vi "SCCSup Dialog - GenMCLB.vi"(4 "online help":T1, 6 "filter parameters":T2, 7 "column header strings":string[](array[string]), 9 "listbox selection mode":i32, 10 "dialog title":string, 11 "complete item names":string[][](array[string])) -> (1 "selection":string[][](array[string]), 3 "cancelled?":bool)   [LabVIEW 2020]
uses:
  <vilib>/SourceControl/support/SCCSup Dialog_GenMCLB_FilterParams.ctl
  <vilib>/SourceControl/support/SCCSup Dialog_GenMCLB_OnlineHelp.ctl
  <vilib>/event_ctls.llb/sizeaction.ctl
  <vilib>/event_ctls.llb/panelstate.ctl
panel:
  out "error out":errorcluster
  in  "error in (no error)":errorcluster
  in  "MC Listbox":i32[](listbox)
  in  "filter":bool=TRUE
  in  "OK":bool
  in  "Cancel":bool
  in  "Help":bool
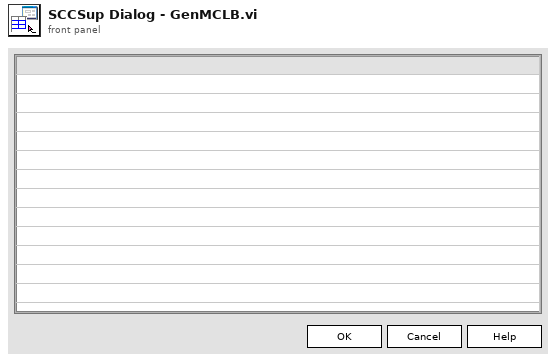
[diagram p1: front panel]
types:
  T1 = typedef "SCCSup Dialog_GenMCLB_OnlineHelp.ctl" = cluster{"Operation":enum16{"Contents", "Key", "Close"}, "String to search for":string, "Path to the help file":path}
  T2 = typedef "SCCSup Dialog_GenMCLB_FilterParams.ctl" = cluster{"checkbox visible?":bool, "boolean text":string, "filter string":string, "filter column":i32}
  T3 = enum32{"invalid OS target", "Mac OS", "Windows 3.1", "Windows 95/NT", "Solaris 1", "Solaris 2", "HP-UX", "PowerMAX", "Linux", "Irix", "Rhapsody", "BeOS", "AIX", "OSF1", "VxWorks", "PharLap", "Carbon", "RTX", "Windows x64", "Linux x64"}
  T4 = typedef "sizeaction.ctl" = enum32{"Minimized", "Maximized", "Resized"}
  T5 = typedef "panelstate.ctl" = enum32{"Standard", "Minimized", "Maximized"}
  T6 = enum32{"Invalid", "Standard", "Closed", "Hidden", "Minimized", "Maximized"}
  T7 = typedef "LVRectTypeDef.ctl" = cluster{"Left":i16, "Top":i16, "Right":i16, "Bottom":i16}
  T8 = enum32{"invalid OS target", "Mac OS", "Windows 3.1", "Windows 95/NT", "Solaris 1", "Solaris 2", "HP-UX", "PowerMAX", "Linux", "Irix", "Rhapsody", "BeOS", "AIX", "OSF1", "VxWorks", "PharLap", "Carbon", "RTX", "Windows x64", "Linux x64", "Mac OS X x64"}
  T9 = typedef "LVPoint32TypeDef.ctl" = cluster{"Horizontal":i32, "Vertical":i32}
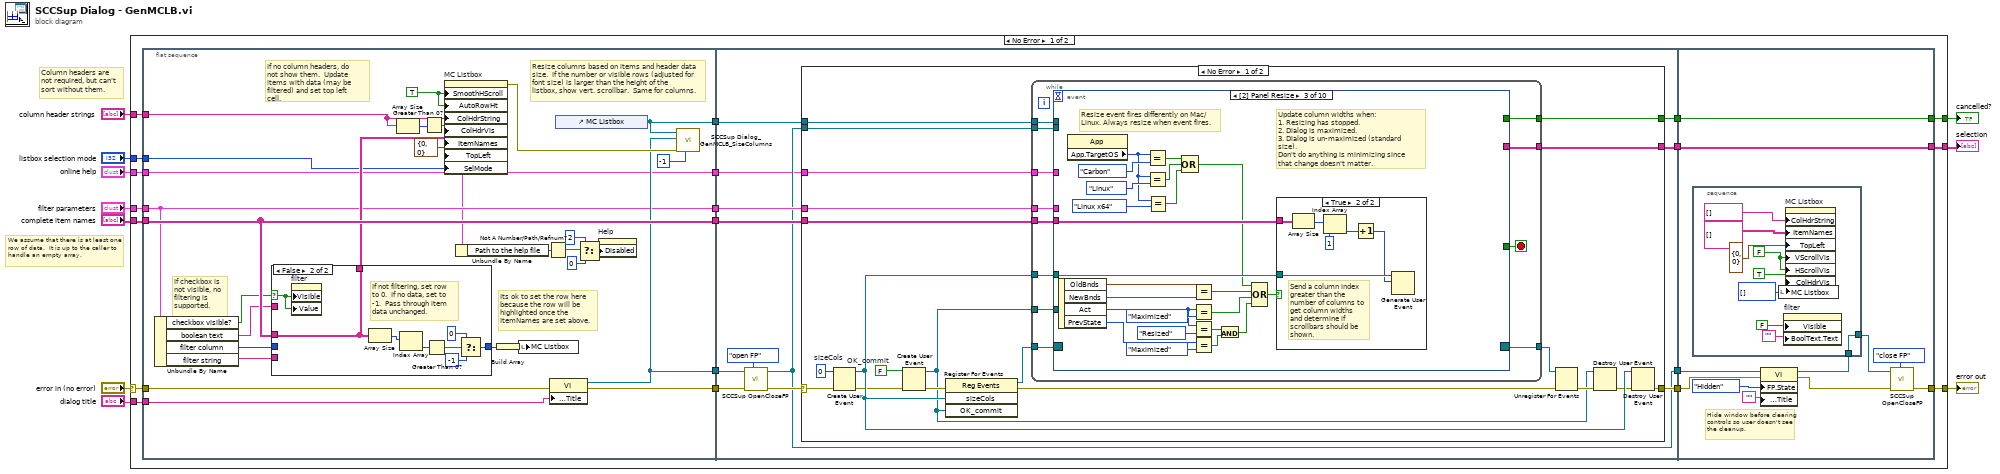
[diagram p0: block diagram]
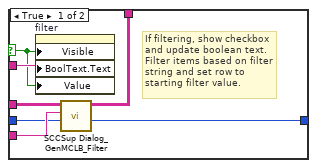
[diagram p2: hidden frame]
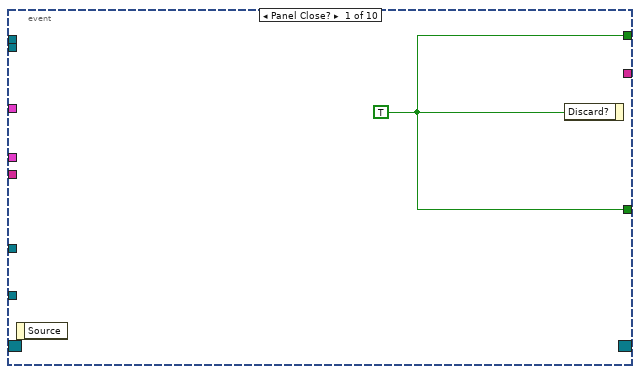
[diagram p3: hidden frame]
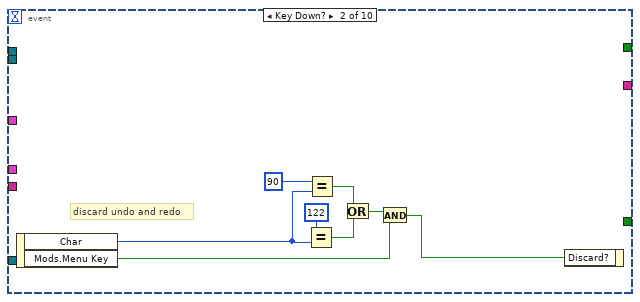
[diagram p4: hidden frame]
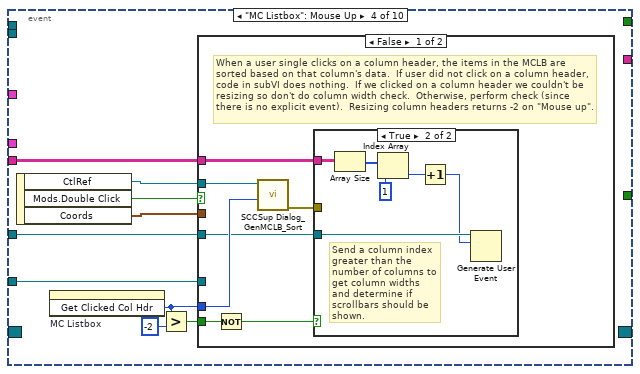
[diagram p6: hidden frame]
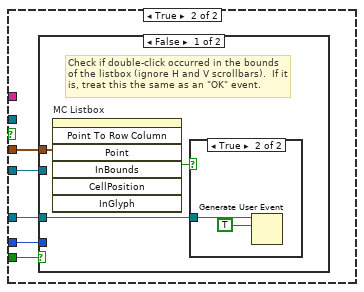
[diagram p8: hidden frame]
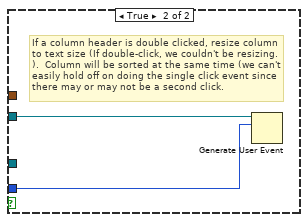
[diagram p10: hidden frame]
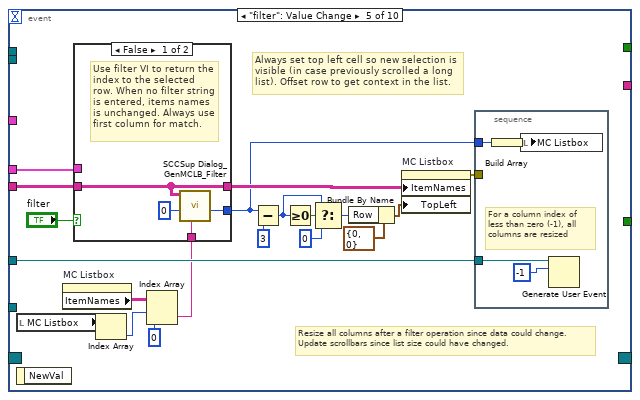
[diagram p11: hidden frame]
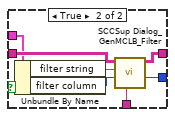
[diagram p12: hidden frame]
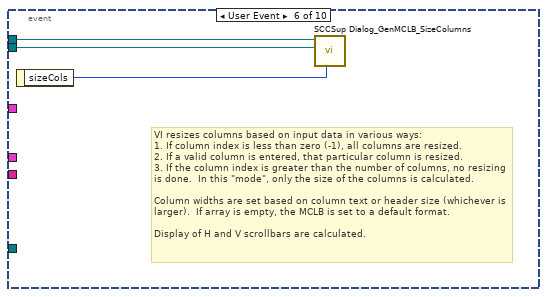
[diagram p13: hidden frame]
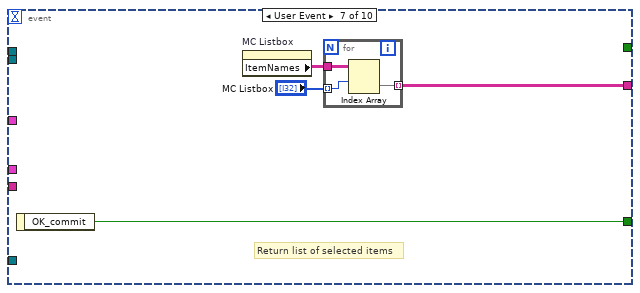
[diagram p14: hidden frame]
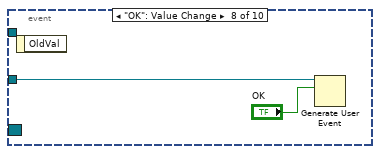
[diagram p15: hidden frame]
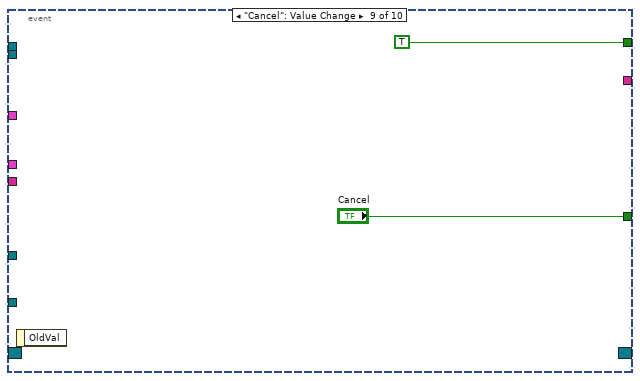
[diagram p16: hidden frame]
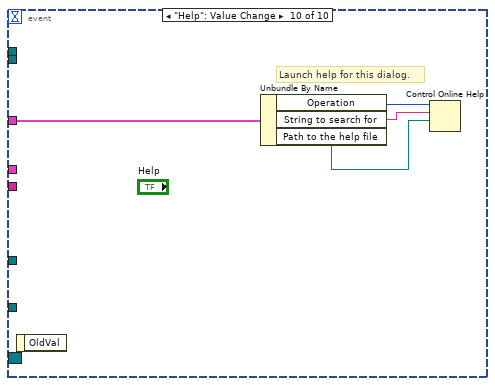
[diagram p17: hidden frame]
diagram:
  # "Column headers are not required, but can't sort without them."
  # "We assume that there is at least one row of data.  It is up to the caller to handle an empty array."
  n1 = case shown="No Error" "error in (no error)" {
    selector: "error in (no error)" -> [w16 w263]
    tunnel: "dialog title" -> [w23 _]
    tunnel: "complete item names" -> [w22 _]
    tunnel: "column header strings" -> [w21 _]
    tunnel: "filter parameters" -> [w20 _]
    tunnel: "listbox selection mode" -> [w19 _]
    tunnel: [w18 _] -> w5
    tunnel: [w17 _] -> w4
    tunnel: [w13 w263] -> w2
    tunnel: "online help" -> [w12 _]
    frame No Error {
      n2 = flat-sequence {
        tunnel: [w45] -> w30
        tunnel: w23 -> [w58]
        tunnel: w22 -> [w53]
        tunnel: w21 -> [w54]
        tunnel: [w53] -> w29
        tunnel: w20 -> [w41]
        tunnel: [w41] -> w28
        tunnel: [w47] -> w27
        tunnel: w19 -> [w46]
        tunnel: w16 -> [w44]
        tunnel: [w43] -> w15
        tunnel: w12 -> [w36]
        tunnel: [w36] -> w11
        tunnel: [w75] -> w26
        tunnel: w30 -> [w84]
        tunnel: w29 -> [w83]
        tunnel: w28 -> [w82]
        tunnel: w27 -> [w81]
        tunnel: [w80] -> w25
        tunnel: [w79] -> w24
        tunnel: w15 -> [w78]
        tunnel: [w76] -> w14
        tunnel: w11 -> [w74]
        tunnel: w26 -> [w253]
        tunnel: [w251] -> w18
        tunnel: w25 -> [w251]
        tunnel: [w250] -> w17
        tunnel: w24 -> [w250]
        tunnel: w14 -> [w249]
        tunnel: [w247] -> w13
        frame #0 {
          w42 = TRUE ("Smooth Horizontal Scrolling")
          # "If checkbox is not visible, no filtering is supported."
          # "Resize columns based on items and header data size.  If the number or visible rows (adjusted for font size) is larger than the height of the listbox, show vert. scrollbar.  Same for columns."
          # "Its ok to set the row here because the row will be highlighted once the ItemNames are set above."
          # "If no column headers, do not show them.  Update items with data (may be filtered) and set top left cell."
          n3 = Unbundle By Name(w41) -> ("checkbox visible?"=w40:bool, "boolean text"=w39:string, "filter column"=w38:i32, "filter string"=w37:string)
          n4 = case shown="False" w40 {
            selector: w40 -> [w59 w66]
            tunnel: w39 -> [w65 _]
            tunnel: w53 -> [w64 w68]
            tunnel: w38 -> [w61 _]
            tunnel: w37 -> [w62 _]
            tunnel: [w60 w69] -> w57
            tunnel: [w63 w68] -> w51
            frame True {
              # "If filtering, show checkbox and update boolean text.  Filter items based on filter string and set row to starting filter value."
              n5 = property on="filter" class="Bool (strict)"("Visible"=w59, "BoolText.Text"=w65, "Value"=w59) -> ()  [unwired: 2 in, 2 out]
              n6 = call <vilib>:"SCCSup Dialog_GenMCLB_Filter.vi"("filter column"=w61, "filter string"=w62, "complete item names"=w64) -> ("filter string row index"=w60:i32, "filtered item names"=w63:string[][])  [unwired: 7 in]
            }
            frame False {
              # "If not filtering, set row to 0.  If no data, set to -1.  Pass through item data unchanged."
              n7 = property on="filter" class="Bool (strict)"("Visible"=w66, "Value"=w66) -> ()  [unwired: 2 in, 2 out]
              n8 = Array Size(array=w68) -> (size(s)=w73:i32[])
              n9 = Index Array(array=w73) -> (element=w71:i32)  [unwired: 1 in]
              n10 = Greater Than 0?(x=w71) -> (x > 0?=w72:bool)
              n11 = Select(t=0, s=w72, f=-1 ("index of element")) -> (s? t:f=w69:i32)
            }
          }
          n12 = Array Size(array=w54) -> (size(s)=w56:i32)
          n13 = Greater Than 0?(x=w56) -> (x > 0?=w55:bool)
          n14 = property on="MC Listbox" class="MCListbox (strict)"("SmoothHScroll"=w42, "AutoRowHt"=w42, "ColHdrString"=w54, "ColHdrVis"=w55, "ItemNames"=w51, "TopLeft"=cluster{"Row":u32, "Column":u32} {"Row"=0, "Column"=0} ("Top Left Visible Cell"), "SelMode"=w46) -> (error out=w49:errorcluster)  [unwired: 2 in, 1 out]
          n15 = Unbundle By Name(w36) -> ("Path to the help file"=w35:path)
          n16 = Build Array(w57) -> (w48:i32[])
          n17 = local write "MC Listbox"(w48) -> ()
          n18 = Not A Number/Path/Refnum?(number/path/refnum=w35) -> (NaN/Path/Refnum?=w34:bool)
          n19 = property class="VI"(error in=w44, "Front Panel.Title"=w58) -> (reference out=w45:refnum<vi>, error out=w43:errorcluster)  [unwired: 1 in]
          n20 = control-ref of="MC Listbox"() -> (w47:refnum<vi>)
          n21 = Select(t=u8 2 ("Disabled"), s=w34, f=u8 0 ("Disabled")) -> (s? t:f=w31:u8)
          n22 = property on="Help" class="Bool"("Disabled"=w31) -> ()  [unwired: 2 in, 2 out]
          n23 = call <vilib>:"SCCSup Dialog_GenMCLB_SizeColumns.vi"("column index"=-1, "error in (no error)"=w49, "VI Refnum"=w45, "Multicolumn Listbox"=w47) -> ()  [unwired: 6 in, 2 out]
        }
        frame #1 {
          n24 = call <vilib>:"SCCSup OpenCloseFP.vi"("function"=enum16{"open FP", "close FP"}."open FP", "error in (no error)"=w78, "VI Refnum in"=w84) -> ("error out"=w77:errorcluster, "VI Refnum out"=w75:refnum<vi>)  [unwired: 7 in]
          n25 = case shown="No Error" w77 {
            selector: w77 -> [w100 w242]
            tunnel: w75 -> [w94 _]
            tunnel: w83 -> [w105 _]
            tunnel: w82 -> [w104 _]
            tunnel: w81 -> [w103 _]
            tunnel: [w102 _] -> w80
            tunnel: [w101 _] -> w79
            tunnel: [w95 w242] -> w76
            tunnel: w74 -> [w86 _]
            frame No Error {
              w90 = FALSE  # OK_commit
              w93 = 0  # sizeCols
              n26 = Create User Event(user event datatype=w93, error in=w100) -> (user event=w96:refnum<user-event>, error out=w91:errorcluster)
              n27 = Create User Event(user event datatype=w90, error in=w91) -> (user event=w87:refnum<user-event>, error out=w92:errorcluster)
              n28 = register-events(error in=w92, w96, w87) -> (reference out=w99:refnum<event-registration>, error out=w98:errorcluster)  [unwired: 1 in]
              n29 = while {
                tunnel: [w116] -> w102
                tunnel: w94 -> [w111]
                tunnel: [w115] -> w101
                tunnel: w105 -> [w114]
                tunnel: w104 -> [w113]
                tunnel: w103 -> [w112]
                tunnel: w96 -> [w108]
                tunnel: w99 -> [w110]
                tunnel: [w109] -> w97
                tunnel: w87 -> [w107]
                tunnel: w86 -> [w106]
                stop <- w117 stop-if-true
                n30 = event shown="[2] Panel Resize" {
                  selector: w110 -> [_ _ _ _ _ _ _ _ _ _]
                  dyn-events: [_ _ _ _ _ _ _ _ _ _] -> w109
                  timeout: _ -> [_ _ _ _ _ _ _ _ _ _]
                  tunnel: [w118 _ _ _ _ _ w227 _ "Cancel" _] -> w117
                  tunnel: [w118 _ _ _ _ _ _ _ TRUE _] -> w116
                  tunnel: [_ _ _ _ _ _ w228 _ _ _] -> w115
                  tunnel: w114 -> [_ _ w136 w159 w208 _ _ _ _ _]
                  tunnel: w113 -> [_ _ _ _ w206 _ _ _ _ _]
                  tunnel: w112 -> [_ _ _ _ _ w226 _ _ _ _]
                  tunnel: w111 -> [_ _ _ _ _ w225 _ _ _ _]
                  tunnel: w108 -> [_ _ w137 w158 w204 _ _ _ _ _]
                  tunnel: w107 -> [_ _ _ w157 _ _ _ w235 _ _]
                  tunnel: w106 -> [_ _ _ _ _ _ _ _ _ w238]
                  event Panel Close? {
                    w118 = TRUE
                    n31 = event-data() -> ()  [unwired: 1 in, 1 out]
                    n32 = event-data("Discard?"=w118) -> ()  [unwired: 1 in, 1 out]
                  }
                  event Key Down? {
                    # "discard undo and redo"
                    n33 = event-data() -> ("Char"=w121:i16, "Mods.Menu Key"=w120:bool)  [unwired: 1 in]
                    n34 = Equal?(x=i16 122, y=w121) -> (x = y?=w124:bool)
                    n35 = Equal?(x=i16 90, y=w121) -> (x = y?=w123:bool)
                    n36 = Or(x=w123, y=w124) -> (x .or. y?=w122:bool)
                    n37 = And(x=w122, y=w120) -> (x .and. y?=w119:bool)
                    n38 = event-data("Discard?"=w119) -> ()  [unwired: 1 in, 1 out]
                  }
                  event Panel Resize {
                    # "Resize event fires differently on Mac/Linux. Always resize when event fires."
                    # "Update column widths when:\n1. Resizing has stopped.\n2. Dialog is maximized.\n3. Dialog is un-maximized (standard size).\nDon't do anything is minimizing since that change doesn't matter."
                    n39 = event-data() -> ("OldBnds"=w149:T7, "NewBnds"=w148:T7, "Act"=w142:T4, "PrevState"=w144:T5)  [unwired: 1 in]
                    n40 = property class="App"() -> ("App.TargetOS"=w129:T8)  [unwired: 2 in, 2 out]
                    n41 = Equal?(x=w129, y=T3."Carbon" ("Application:Target:Operating System")) -> (x = y?=w135:bool)
                    n42 = Equal?(x=w129, y=T3."Linux" ("Application:Target:Operating System")) -> (x = y?=w130:bool)
                    n43 = Equal?(x=w129, y=T3."Linux x64" ("Application:Target:Operating System")) -> (x = y?=w127:bool)
                    n44 = Compound Arithmetic op=OR(w135, w130, w127) -> (w134:bool)
                    n45 = Equal?(x=w149, y=w148) -> (x = y?=w133:bool)
                    n46 = Equal?(x=w142, y=sizeaction."Maximized") -> (x = y?=w145:bool)
                    n47 = Equal?(x=w142, y=sizeaction."Resized") -> (x = y?=w140:bool)
                    n48 = Equal?(x=w144, y=panelstate."Maximized" ("PrevState")) -> (x = y?=w139:bool)
                    n49 = And(x=w140, y=w139) -> (x .and. y?=w138:bool)
                    n50 = Compound Arithmetic op=OR(w134, w133, w145, w138) -> (w146:bool)
                    n51 = case shown="True" w146 {
                      tunnel: w137 -> [_ w155]
                      tunnel: w136 -> [_ w151]
                      frame False {
                      }
                      frame True {
                        # "Send a column index greater than the number of columns to get column widths and determine if scrollbars should be shown."
                        n52 = Array Size(array=w151) -> (size(s)=w153:i32[])
                        n53 = Index Array(array=w153, index=1) -> (element=w154:i32)
                        n54 = Increment(x=w154) -> (x+1=w150:i32)
                        n55 = Generate User Event(user event=w155, event data cluster=w150) -> ()  [unwired: 2 in, 2 out]
                      }
                    }
                  }
                  event "MC Listbox": Mouse Up {
                    n56 = event-data() -> ("CtlRef"=w163:refnum<vi>, "Mods.Double Click"=w164:bool, "Coords"=w156:T9)  [unwired: 1 in]
                    n57 = invoke on="MC Listbox" class="MCListbox (strict)" method="Get Clicked Col Hdr"() -> ("Get Clicked Column Header"=w161:i32)  [unwired: 3 in, 2 out]
                    n58 = Greater?(x=w161, y=-2) -> (0:w160:bool)
                    n59 = case shown="False" w164 {
                      tunnel: w163 -> [w169 _]
                      tunnel: w161 -> [w171 w182]
                      tunnel: w160 -> [w170 w181]
                      tunnel: w159 -> [w168 _]
                      tunnel: w158 -> [w166 w180]
                      tunnel: w157 -> [_ w179]
                      tunnel: w156 -> [_ w178]
                      frame False {
                        # "When a user single clicks on a column header, the items in the MCLB are sorted based on that column's data.  If user did not click on a column header, code in subVI does nothing.  If we clicked on a column header we couldn't be resizing so don't do column width check.  Otherwise, perform check (since there is no explicit event).  Resizing column headers returns -2 on \"Mouse up\"."
                        n60 = Not(x=w170) -> (.not. x?=w167:bool)
                        n61 = call <vilib>:"SCCSup Dialog_GenMCLB_Sort.vi"("Clicked Col Hdr"=w171, "MCListbox Refnum"=w169) -> ("error out"=w165:errorcluster)  [unwired: 9 in]
                        n62 = case shown="True" w167 {
                          tunnel: w168 -> [_ w177]
                          tunnel: w166 -> [_ w173]
                          tunnel: w165 -> [_ _]
                          frame False {
                          }
                          frame True {
                            # "Send a column index greater than the number of columns to get column widths and determine if scrollbars should be shown."
                            n63 = Array Size(array=w177) -> (size(s)=w175:i32[])
                            n64 = Index Array(array=w175, index=1) -> (element=w174:i32)
                            n65 = Increment(x=w174) -> (x+1=w172:i32)
                            n66 = Generate User Event(user event=w173, event data cluster=w172) -> ()  [unwired: 2 in, 2 out]
                          }
                        }
                      }
                      frame True {
                        n67 = case shown="False" w181 {
                          tunnel: w182 -> [_ w188]
                          tunnel: w180 -> [_ w189]
                          tunnel: w179 -> [w183 _]
                          tunnel: w178 -> [w185 _]
                          frame False {
                            # "Check if double-click occurred in the bounds of the listbox (ignore H and V scrollbars).  If it is, treat this the same as an \"OK\" event."
                            n68 = invoke on="MC Listbox" class="MCListbox (strict)" method="Point To Row Column"("Point"=w185) -> ("InBounds"=w184:bool)  [unwired: 6 in, 6 out]
                            n69 = case shown="True" w184 {
                              tunnel: w183 -> [_ w187]
                              frame False {
                              }
                              frame True {
                                n70 = Generate User Event(user event=w187, event data cluster=TRUE ("event data")) -> ()  [unwired: 2 in, 2 out]
                              }
                            }
                          }
                          frame True {
                            # "If a column header is double clicked, resize column to text size (If double-click, we couldn't be resizing.).  Column will be sorted at the same time (we can't easily hold off on doing the single click event since there may or may not be a second click."
                            n71 = Generate User Event(user event=w189, event data cluster=w188) -> ()  [unwired: 2 in, 2 out]
                          }
                        }
                      }
                    }
                  }
                  event "filter": Value Change {
                    # "Always set top left cell so new selection is visible (in case previously scrolled a long list). Offset row to get context in the list."
                    # "Resize all columns after a filter operation since data could change.  Update scrollbars since list size could have changed."
                    n72 = local read "MC Listbox"() -> (w196:i32[])
                    n73 = event-data() -> ()  [unwired: 1 in, 1 out]
                    n74 = property on="MC Listbox" class="MCListbox (strict)"() -> ("ItemNames"=w197:string[][])  [unwired: 2 in, 2 out]
                    n75 = Index Array(array=w196) -> (element=w195:i32)  [unwired: 1 in]
                    n76 = Index Array(array=w197, index (row)=w195, index (col)=0 ("disabled index (col)")) -> (element=w193:string)
                    n77 = case shown="False" "filter" {
                      tunnel: w208 -> [w214 w223]
                      tunnel: [w214 w222] -> w207
                      tunnel: [w215 w221] -> w192
                      tunnel: w206 -> [_ w220]
                      tunnel: w193 -> [w216 w217]
                      frame False {
                        # "Use filter VI to return the index to the selected row. When no filter string is entered, items names is unchanged. Always use first column for match."
                        n78 = call <vilib>:"SCCSup Dialog_GenMCLB_Filter.vi"("current selection"=w216, "filter column"=0, "complete item names"=w214) -> ("filter string row index"=w215:i32)  [unwired: 7 in, 1 out]
                      }
                      frame True {
                        n79 = Unbundle By Name(w220) -> ("filter string"=w219:string, "filter column"=w218:i32)
                        n80 = call <vilib>:"SCCSup Dialog_GenMCLB_Filter.vi"("current selection"=w217, "filter column"=w218, "filter string"=w219, "complete item names"=w223) -> ("filter string row index"=w221:i32, "filtered item names"=w222:string[][])  [unwired: 6 in]
                      }
                    }
                    n81 = Subtract(x=w192, y=3) -> (x-y=w190:i32)
                    n82 = Greater Or Equal To 0?(x=w190) -> (x >= 0?=w203:bool)
                    n83 = Select(t=w190, s=w203, f=0 ("y")) -> (s? t:f=w200:i32)
                    n84 = Bundle By Name(cluster=cluster{"Row":u32, "Column":u32} {"Row"=0, "Column"=0} ("Top Left Visible Cell"), "Row"=w200) -> (w199:cluster{"Row":u32, "Column":u32})
                    n85 = property on="MC Listbox" class="MCListbox (strict)"("ItemNames"=w207, "TopLeft"=w199) -> (error out=w198:errorcluster)  [unwired: 2 in, 1 out]
                    n86 = stacked-sequence {
                      tunnel: w204 -> [w211]
                      tunnel: w198 -> [_]
                      tunnel: w192 -> [w209]
                      frame #0 {
                        # "For a column index of less than zero (-1), all columns are resized"
                        n87 = Build Array(w209) -> (w212:i32[])
                        n88 = local write "MC Listbox"(w212) -> ()
                        n89 = Generate User Event(user event=w211, event data cluster=-1 ("column index")) -> ()  [unwired: 2 in, 2 out]
                      }
                    }
                  }
                  event User Event {
                    # "VI resizes columns based on input data in various ways:\n1. If column index is less than zero (-1), all columns are resized.\n2. If a valid column is entered, that particular column is resized.\n3. If the column index is greater than the number of columns, no resizing is done.  In this \"mode\", only the size of the columns is calculated.\n\nColumn widths are set based on column text or header size (whichever is larger).  If array is empty, the MCLB is set to a default format.\n\nDisplay of H and V scrollbars are calculated."
                    n90 = event-data() -> ("sizeCols"=w224:i32)  [unwired: 1 in]
                    n91 = call <vilib>:"SCCSup Dialog_GenMCLB_SizeColumns.vi"("column index"=w224, "VI Refnum"=w225, "Multicolumn Listbox"=w226) -> ()  [unwired: 7 in, 2 out]
                  }
                  event User Event {
                    # "Return list of selected items"
                    n92 = event-data() -> ("OK_commit"=w227:bool)  [unwired: 1 in]
                    n93 = property on="MC Listbox" class="MCListbox (strict)"() -> ("ItemNames"=w230:string[][])  [unwired: 2 in, 2 out]
                    n94 = for {
                      tunnel: w230 -> [w233]
                      tunnel: [w232] -> w228 mode=indexing
                      tunnel: "MC Listbox" -> [w231] mode=indexing
                      n95 = Index Array(array=w233, index (row)=w231) -> (element=w232:string[])  [unwired: 1 in]
                    }
                  }
                  event "OK": Value Change {
                    n96 = event-data() -> ()  [unwired: 1 in, 1 out]
                    n97 = Generate User Event(user event=w235, event data cluster="OK") -> ()  [unwired: 2 in, 2 out]
                  }
                  event "Cancel": Value Change {
                    n98 = event-data() -> ()  [unwired: 1 in, 1 out]
                  }
                  event "Help": Value Change {
                    # "Launch help for this dialog."
                    n99 = event-data() -> ()  [unwired: 1 in, 1 out]
                    n100 = Unbundle By Name(w238) -> ("Operation"=w241:enum16{"Contents", "Key", "Close"}, "String to search for"=w240:string, "Path to the help file"=w239:path)
                    n101 = Control Online Help(2:w239, 3:w240, 4:w241) -> ()  [unwired: 1 in, 1 out]
                  }
                }
              }
              n102 = Unregister For Events(event registration refnum=w97, error in=w98) -> (error out=w88:errorcluster)
              n103 = Destroy User Event(user event=w87, error in=w88) -> (error out=w89:errorcluster)
              n104 = Destroy User Event(user event=w96, error in=w89) -> (error out=w95:errorcluster)
            }
            frame Error {
            }
          }
        }
        frame #2 {
          # "Hide window before clearing controls so user doesn't see the cleanup."
          n105 = property class="VI"(reference=w253, error in=w249, "FP.State"=T6."Hidden" ("Front Panel Window:State"), "Front Panel.Title"="") -> (reference out=w244:refnum<vi>, error out=w248:errorcluster)
          n106 = stacked-sequence {
            tunnel: [w254] -> w243
            tunnel: w244 -> [w254]
            frame #0 {
              w259 = FALSE ("Vertical Scrollbar Visible")
              n107 = local write "MC Listbox"(i32[] [] ("MC Listbox")) -> ()
              n108 = property on="filter" class="Bool (strict)"("Visible"=FALSE, "BoolText.Text"="") -> ()  [unwired: 2 in, 2 out]
              n109 = property on="MC Listbox" class="MCListbox (strict)"("ColHdrString"=string[] [] ("Column Header Strings"), "ItemNames"=string[][] [] ("Item Names"), "TopLeft"=cluster{"Row":u32, "Column":u32} {"Row"=0, "Column"=0} ("Top Left Visible Cell"), "VScrollVis"=w259, "HScrollVis"=w259, "ColHdrVis"=TRUE ("Column Headers Visible")) -> ()  [unwired: 2 in, 2 out]
            }
          }
          n110 = call <vilib>:"SCCSup OpenCloseFP.vi"("function"=enum16{"open FP", "close FP"}."close FP", "error in (no error)"=w248, "VI Refnum in"=w243) -> ("error out"=w247:errorcluster)  [unwired: 7 in, 1 out]
        }
      }
    }
    frame Error {
    }
  }
  "cancelled?" <- w5
  "selection" <- w4
  "error out" <- w2
